vi "Decode.vi"(7 "Variant (Base64)":T1, 8 "error in (no error)":errorcluster, 10 "string in (base64-encoded)":string) -> (0 "error out":errorcluster, 2 "string out (decoded)":string)   [LabVIEW 2020, in "Base64.lvlib"]
doc: "Decodes a Base64 encoded string, optionally from the Base64-URL variant."
uses:
  Base64.lvlib
  Variant.ctl
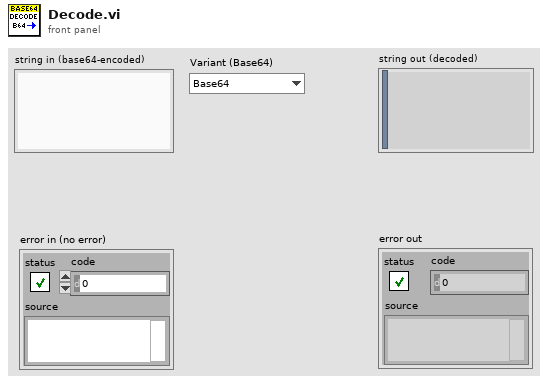
[diagram p1: front panel]
types:
  T1 = typedef "Base64.lvlib/Variant.ctl" = enum16{"Base64", "Base64-URL"}
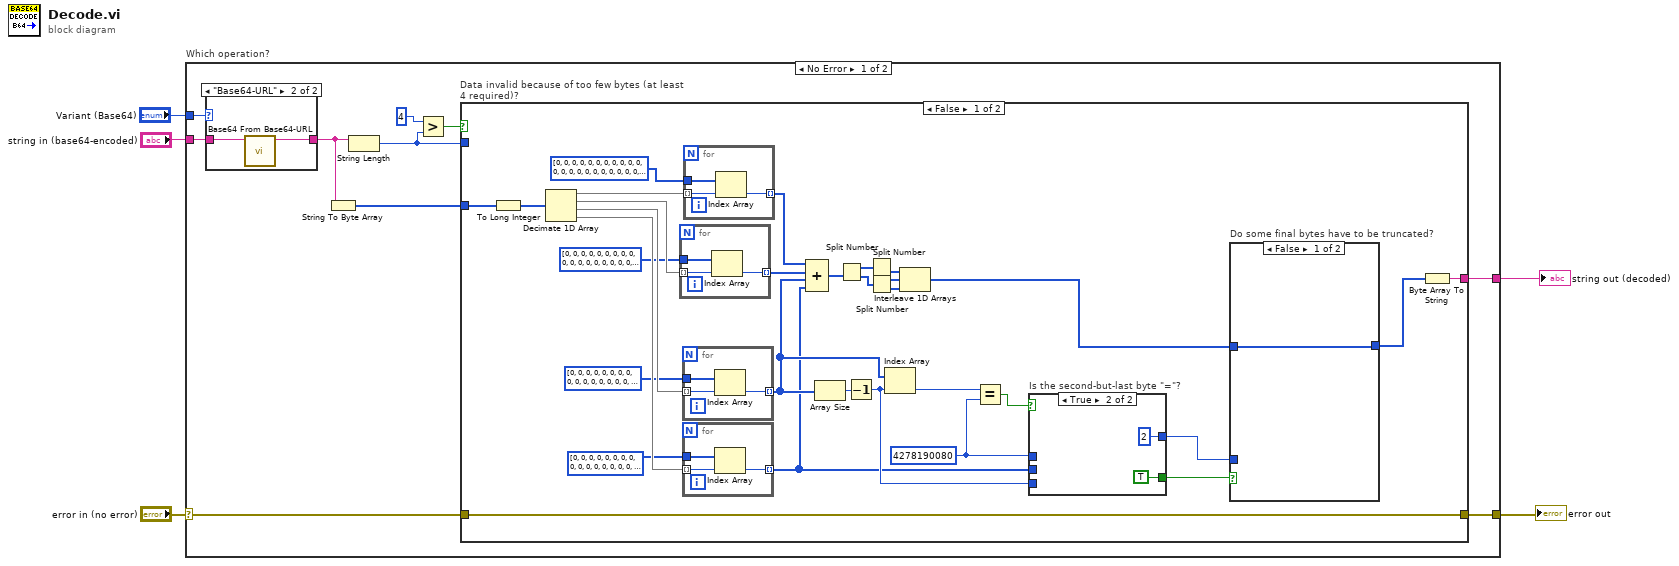
[diagram p0: block diagram]
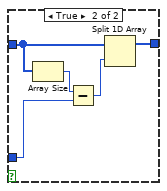
[diagram p3: hidden frame]
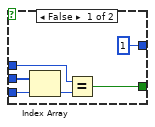
[diagram p4: hidden frame]
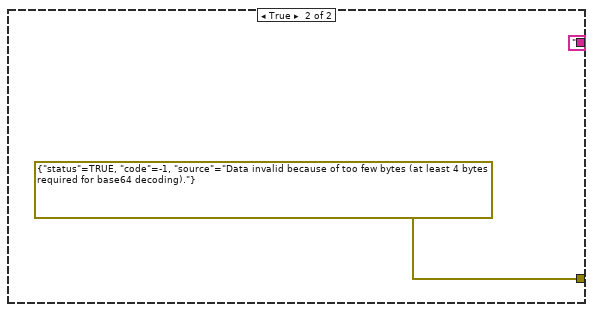
[diagram p5: hidden frame]
diagram:
  n1 = case "Which operation?" shown="No Error" "error in (no error)" {
    selector: "error in (no error)" -> [w13 w78]
    tunnel: "string in (base64-encoded)" -> [w7 _]
    tunnel: [w12 w78] -> w4
    tunnel: [w11 _] -> w2
    tunnel: "Variant (Base64)" -> [w8 _]
    frame No Error {
      n2 = case shown="\"Base64-URL\"" w8 {
        tunnel: w7 -> [w16 w18]
        tunnel: [w16 w17] -> w6
        frame "Base64" {
        }
        frame "Base64-URL" {
          n3 = call "Base64 From Base64-URL.vi"("Base64-URL String"=w18) -> ("Base64 String"=w17:string)  [unwired: 10 in]
        }
      }
      n4 = String To Byte Array(string=w6) -> (unsigned byte array=w15:u8[])
      n5 = String Length(string=w6) -> (length=w10:i32)
      n6 = Greater?(x=4 ("y"), y=w10) -> (0:w14:bool)
      n7 = case "Data invalid because of too few bytes (at least 4 required)?" shown="False" w14 {
        tunnel: w15 -> [w31 _]
        tunnel: [w49 ""] -> w11
        tunnel: w10 -> [_ _]
        tunnel: [w23 errorcluster {"status"=TRUE, "code"=-1, "source"="Data invalid because of too few bytes (at least 4 bytes required for base64 decoding)."} ("error IO")] -> w12
        tunnel: w13 -> [w23 _]
        frame False {
          w24 = u32 4278190080 ("y")
          n8 = To Long Integer(number=w31) -> (32bit integer=w48:i32[])
          n9 = Decimate 1D Array(w48) -> (w37:i32[], w47:i32[], w38:i32[], w36:i32[])
          n10 = for {
            tunnel: w47 -> [w57] mode=indexing
            tunnel: u32[] [0, 0, 0, 0, 0, 0, 0, 0, 0, 0, 0, 0, 0, 0, 0, 0, 0, 0, 0, 0, 0, 0, 0, 0, 0, 0, 0, 0, 0, 0, 0, 0, 0, 0, 0, 0, 0, 0, 0, 0, 0, 0, 0, 253952, 0, 0, 0, 258048, 212992, 217088, 221184, 225280, 229376, 233472, 237568, 241664, 245760, 249856, 0, 0, 0, 0, 0, 0, 0, 0, 4096, 8192, 12288, 16384, 20480, 24576, 28672, 32768, 36864, 40960, 45056, 49152, 53248, 57344, 61440, 65536, 69632, 73728, 77824, 81920, 86016, 90112, 94208, 98304, 102400, 0, 0, 0, 0, 0, 0, 106496, 110592, 114688, 118784, 122880, 126976, 131072, 135168, 139264, 143360, 147456, 151552, 155648, 159744, 163840, 167936, 172032, 176128, 180224, 184320, 188416, 192512, 196608, 200704, 204800, 208896, 0, 0, 0, 0, 0, 0, 0, 0, 0, 0, 0, 0, 0, 0, 0, 0, 0, 0, 0, 0, 0, 0, 0, 0, 0, 0, 0, 0, 0, 0, 0, 0, 0, 0, 0, 0, 0, 0, 0, 0, 0, 0, 0, 0, 0, 0, 0, 0, 0, 0, 0, 0, 0, 0, 0, 0, 0, 0, 0, 0, 0, 0, 0, 0, 0, 0, 0, 0, 0, 0, 0, 0, 0, 0, 0, 0, 0, 0, 0, 0, 0, 0, 0, 0, 0, 0, 0, 0, 0, 0, 0, 0, 0, 0, 0, 0, 0, 0, 0, 0, 0, 0, 0, 0, 0, 0, 0, 0, 0, 0, 0, 0, 0, 0, 0, 0, 0, 0, 0, 0, 0, 0, 0, 0, 0, 0, 0, 0, 0, 0, 0, 0, 0] ("array 3") -> [w58]
            tunnel: [w56] -> w45 mode=indexing
            n11 = Index Array(array=w58, index=w57) -> (element=w56:u32)
          }
          n12 = for {
            tunnel: u32[] [0, 0, 0, 0, 0, 0, 0, 0, 0, 0, 0, 0, 0, 0, 0, 0, 0, 0, 0, 0, 0, 0, 0, 0, 0, 0, 0, 0, 0, 0, 0, 0, 0, 0, 0, 0, 0, 0, 0, 0, 0, 0, 0, 3968, 0, 0, 0, 4032, 3328, 3392, 3456, 3520, 3584, 3648, 3712, 3776, 3840, 3904, 0, 0, 0, 4278190080, 0, 0, 0, 0, 64, 128, 192, 256, 320, 384, 448, 512, 576, 640, 704, 768, 832, 896, 960, 1024, 1088, 1152, 1216, 1280, 1344, 1408, 1472, 1536, 1600, 0, 0, 0, 0, 0, 0, 1664, 1728, 1792, 1856, 1920, 1984, 2048, 2112, 2176, 2240, 2304, 2368, 2432, 2496, 2560, 2624, 2688, 2752, 2816, 2880, 2944, 3008, 3072, 3136, 3200, 3264, 0, 0, 0, 0, 0, 0, 0, 0, 0, 0, 0, 0, 0, 0, 0, 0, 0, 0, 0, 0, 0, 0, 0, 0, 0, 0, 0, 0, 0, 0, 0, 0, 0, 0, 0, 0, 0, 0, 0, 0, 0, 0, 0, 0, 0, 0, 0, 0, 0, 0, 0, 0, 0, 0, 0, 0, 0, 0, 0, 0, 0, 0, 0, 0, 0, 0, 0, 0, 0, 0, 0, 0, 0, 0, 0, 0, 0, 0, 0, 0, 0, 0, 0, 0, 0, 0, 0, 0, 0, 0, 0, 0, 0, 0, 0, 0, 0, 0, 0, 0, 0, 0, 0, 0, 0, 0, 0, 0, 0, 0, 0, 0, 0, 0, 0, 0, 0, 0, 0, 0, 0, 0, 0, 0, 0, 0, 0, 0, 0, 0, 0, 0, 0] ("array 2") -> [w75]
            tunnel: [w74] -> w29 mode=indexing
            tunnel: w38 -> [w73] mode=indexing
            n13 = Index Array(array=w75, index=w73) -> (element=w74:u32)
          }
          n14 = for {
            tunnel: u32[] [0, 0, 0, 0, 0, 0, 0, 0, 0, 0, 0, 0, 0, 0, 0, 0, 0, 0, 0, 0, 0, 0, 0, 0, 0, 0, 0, 0, 0, 0, 0, 0, 0, 0, 0, 0, 0, 0, 0, 0, 0, 0, 0, 62, 0, 0, 0, 63, 52, 53, 54, 55, 56, 57, 58, 59, 60, 61, 0, 0, 0, 4278190080, 0, 0, 0, 0, 1, 2, 3, 4, 5, 6, 7, 8, 9, 10, 11, 12, 13, 14, 15, 16, 17, 18, 19, 20, 21, 22, 23, 24, 25, 0, 0, 0, 0, 0, 0, 26, 27, 28, 29, 30, 31, 32, 33, 34, 35, 36, 37, 38, 39, 40, 41, 42, 43, 44, 45, 46, 47, 48, 49, 50, 51, 0, 0, 0, 0, 0, 0, 0, 0, 0, 0, 0, 0, 0, 0, 0, 0, 0, 0, 0, 0, 0, 0, 0, 0, 0, 0, 0, 0, 0, 0, 0, 0, 0, 0, 0, 0, 0, 0, 0, 0, 0, 0, 0, 0, 0, 0, 0, 0, 0, 0, 0, 0, 0, 0, 0, 0, 0, 0, 0, 0, 0, 0, 0, 0, 0, 0, 0, 0, 0, 0, 0, 0, 0, 0, 0, 0, 0, 0, 0, 0, 0, 0, 0, 0, 0, 0, 0, 0, 0, 0, 0, 0, 0, 0, 0, 0, 0, 0, 0, 0, 0, 0, 0, 0, 0, 0, 0, 0, 0, 0, 0, 0, 0, 0, 0, 0, 0, 0, 0, 0, 0, 0, 0, 0, 0, 0, 0, 0, 0, 0, 0, 0, 0] ("Array") -> [w72]
            tunnel: [w71] -> w27 mode=indexing
            tunnel: w36 -> [w70] mode=indexing
            n15 = Index Array(array=w72, index=w70) -> (element=w71:u32)
          }
          n16 = for {
            tunnel: w37 -> [w60] mode=indexing
            tunnel: u32[] [0, 0, 0, 0, 0, 0, 0, 0, 0, 0, 0, 0, 0, 0, 0, 0, 0, 0, 0, 0, 0, 0, 0, 0, 0, 0, 0, 0, 0, 0, 0, 0, 0, 0, 0, 0, 0, 0, 0, 0, 0, 0, 0, 16252928, 0, 0, 0, 16515072, 13631488, 13893632, 14155776, 14417920, 14680064, 14942208, 15204352, 15466496, 15728640, 15990784, 0, 0, 0, 0, 0, 0, 0, 0, 262144, 524288, 786432, 1048576, 1310720, 1572864, 1835008, 2097152, 2359296, 2621440, 2883584, 3145728, 3407872, 3670016, 3932160, 4194304, 4456448, 4718592, 4980736, 5242880, 5505024, 5767168, 6029312, 6291456, 6553600, 0, 0, 0, 0, 0, 0, 6815744, 7077888, 7340032, 7602176, 7864320, 8126464, 8388608, 8650752, 8912896, 9175040, 9437184, 9699328, 9961472, 10223616, 10485760, 10747904, 11010048, 11272192, 11534336, 11796480, 12058624, 12320768, 12582912, 12845056, 13107200, 13369344, 0, 0, 0, 0, 0, 0, 0, 0, 0, 0, 0, 0, 0, 0, 0, 0, 0, 0, 0, 0, 0, 0, 0, 0, 0, 0, 0, 0, 0, 0, 0, 0, 0, 0, 0, 0, 0, 0, 0, 0, 0, 0, 0, 0, 0, 0, 0, 0, 0, 0, 0, 0, 0, 0, 0, 0, 0, 0, 0, 0, 0, 0, 0, 0, 0, 0, 0, 0, 0, 0, 0, 0, 0, 0, 0, 0, 0, 0, 0, 0, 0, 0, 0, 0, 0, 0, 0, 0, 0, 0, 0, 0, 0, 0, 0, 0, 0, 0, 0, 0, 0, 0, 0, 0, 0, 0, 0, 0, 0, 0, 0, 0, 0, 0, 0, 0, 0, 0, 0, 0, 0, 0, 0, 0, 0, 0, 0, 0, 0, 0, 0, 0, 0] ("array 4") -> [w61]
            tunnel: [w59] -> w46 mode=indexing
            n17 = Index Array(array=w61, index=w60) -> (element=w59:u32)
          }
          n18 = Compound Arithmetic op=ADD(w46, w45, w29, w27) -> (w43:u32[])
          n19 = Array Size(array=w29) -> (size(s)=w30:i32)
          n20 = Split Number(x=w43) -> (hi(x)=w44:u16[], lo(x)=w42:u16[])
          n21 = Decrement(x=w30) -> (x-1=w28:i32)
          n22 = Split Number(x=w44) -> (lo(x)=w39:u8[])  [unwired: 1 out]
          n23 = Split Number(x=w42) -> (hi(x)=w40:u8[], lo(x)=w41:u8[])
          n24 = Index Array(array=w29, index=w28) -> (element=w26:u32)
          n25 = Interleave 1D Arrays(w39, w40, w41) -> (w22:u8[])
          n26 = Equal?(x=w26, y=w24) -> (x = y?=w25:bool)
          n27 = case "Is the second-but-last byte \"=\"?" shown="True" w25 {
            tunnel: w28 -> [w67 _]
            tunnel: w27 -> [w66 _]
            tunnel: w24 -> [w64 _]
            tunnel: [w63 TRUE] -> w21
            tunnel: [1 2] -> w20
            frame False {
              n28 = Index Array(array=w66, index=w67) -> (element=w65:u32)
              n29 = Equal?(x=w64, y=w65) -> (x = y?=w63:bool)
            }
            frame True {
            }
          }
          n30 = case "Do some final bytes have to be truncated?" shown="False" w21 {
            tunnel: w22 -> [w50 w53]
            tunnel: w20 -> [_ w55]
            tunnel: [w50 w51] -> w19
            frame False {
            }
            frame True {
              n31 = Array Size(array=w53) -> (size(s)=w54:i32)
              n32 = Subtract(x=w54, y=w55) -> (x-y=w52:i32)
              n33 = Split 1D Array(array=w53, index=w52) -> (first subarray=w51:u8[])  [unwired: 1 out]
            }
          }
          n34 = Byte Array To String(unsigned byte array=w19) -> (string=w49:string)
        }
        frame True {
        }
      }
    }
    frame Error {
    }
  }
  "error out" <- w4
  "string out (decoded)" <- w2
